vi "settle-detect-TEST.vi"() -> ()   [LabVIEW 2015]
panel:
  out "Array 3":bool[](array[boolean])
  in  "settled-samples\nthreshold":i16
  in  "error-test-samples":sgl[](array[numeric])
  out "num-settled-samps":i16[](array[numeric])
  in  "error-max":sgl format="%#_13g"
  # "Number of contiguous samples\nthat must be inside the settle boundary\nto consider the trajectory settled"
  # "The settle boundary."
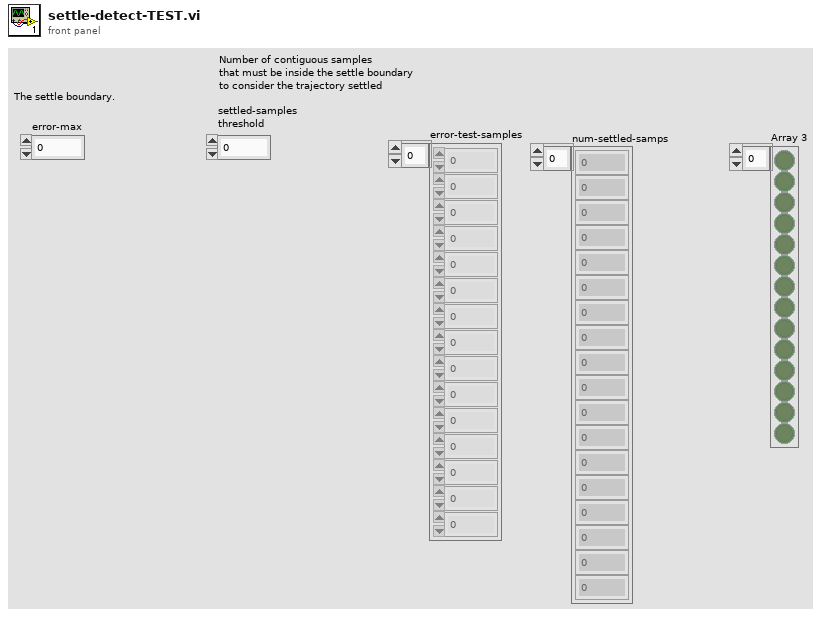
[diagram p1: front panel]
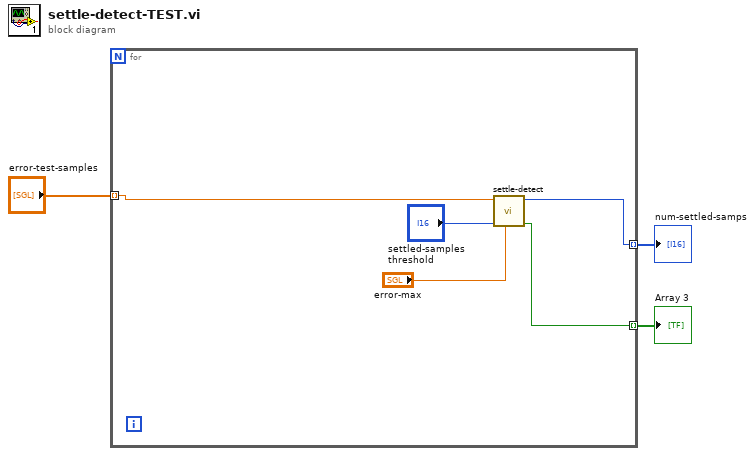
[diagram p0: block diagram]
diagram:
  n1 = for {
    tunnel: [w7] -> w3 mode=indexing
    tunnel: "error-test-samples" -> [w8] mode=indexing
    tunnel: [w4] -> w1 mode=indexing
    n2 = call "settle-detect.vi"("error-max"="error-max", "settled-samples\nthreshold"="settled-samples\nthreshold", "err(k)"=w8) -> ("has-settled"=w4:bool, "number-settled-samples"=w7:i16)  [unwired: 7 in]
  }
  "num-settled-samps" <- w3
  "Array 3" <- w1
